vi "Test Multiplexing.vi"() -> ()   [LabVIEW 2015]
uses:
  Typedefs/HRTF-Hardware Config (TDT).ctl
  PXI DAQ VIs/TDT VIs/Typedefs/TDT-Output source.ctl
  PXI DAQ VIs/TDT VIs/Typedefs/TDT-Device ID.ctl
  PXI DAQ VIs/TDT VIs/Typedefs/TDT-Device Config.ctl
  PXI DAQ VIs/TDT VIs/Typedefs/TDT-Input source.ctl
panel:
  in  "read":bool
  out "GetTagVal":sgl
  in  "stop":bool
  in  "Value":u8=255 format="%08b"
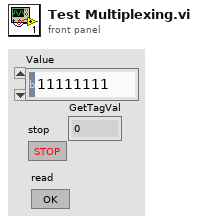
[diagram p1: front panel]
types:
  T1 = typedef "TDT-Device Config.ctl" = cluster{"Output":T2, "Input":T4}
  T2 = typedef "TDT-Output source.ctl" = cluster{"Device":T3, "Num":i32}
  T3 = typedef "TDT-Device ID.ctl" = enum16{"None", "PA5", "RP2", "RL2", "RA16", "RV8", "RX5", "RX6", "RX7", "RX8", "RZ2", "RZ5", "RZ6"}
  T4 = typedef "TDT-Input source.ctl" = enum16{"Front Panel", "RA4LI", "RA16LI"}
  T5 = typedef "HRTF-Hardware Config (TDT).ctl" = cluster{"Output":T2, "Speaker":cluster{"Channel":i32, "Primary mux":i32, "Secondary mux":i32}, "Right mic":i32, "Left mic":i32}
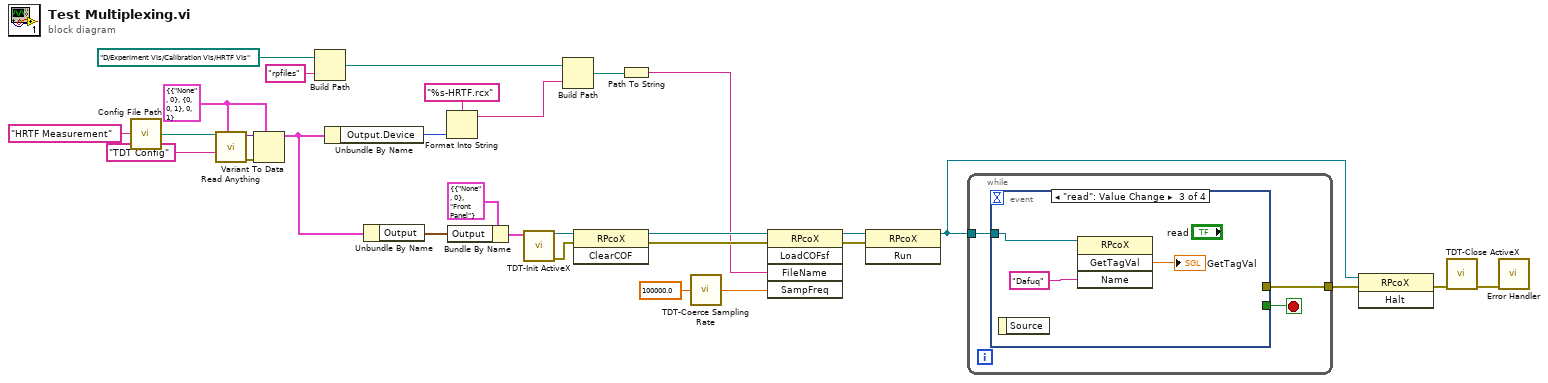
[diagram p0: block diagram]
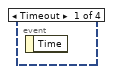
[diagram p2: hidden frame]
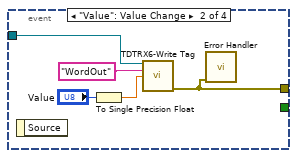
[diagram p3: hidden frame]
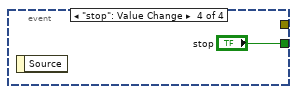
[diagram p4: hidden frame]
diagram:
  w26 = T5 {"Output"={"Device"=enum."None", "Num"=0}, "Speaker"={"Channel"=0, "Primary mux"=0, "Secondary mux"=1}, "Right mic"=0, "Left mic"=1} ("TDT")
  n1 = call "Config File Path.vi"("AppName"="HRTF Measurement") -> ("Default config file name"=w27:path)
  n2 = call "Read Anything.vi"("Type of Anything"=w26, "Section Name (Name of \"Type of Anything\")"="TDT Config" ("Section Name (Name of \"Type of Anything\")"), "Path (dialog)"=w27) -> ("Error Out"=w30:errorcluster, "Anything"=w29:variant)  [unwired: 6 in, 1 out]
  n3 = Variant To Data(error in=w30, type=w26, Variant=w29) -> (data=w21:T5)  [unwired: 1 out]
  n4 = Build Path(base path=path "D:/Experiment VIs/Calibration VIs/HRTF VIs", name or relative path="rpfiles") -> (appended path=w14:path)
  n5 = Unbundle By Name(w21) -> ("Output.Device"=w24:T3)
  n6 = Unbundle By Name(w21) -> ("Output"=w20:T2)
  n7 = Format Into String(format string="%s-HRTF.rcx", w24) -> (resulting string=w12:string)  [unwired: 2 in, 1 out]
  n8 = Bundle By Name(cluster=T1 {"Output"={"Device"=enum."None", "Num"=0}, "Input"=enum."Front Panel"} ("TDT-Device Config"), "Output"=w20) -> (w22:T1)
  n9 = call "TDT-Init ActiveX.vi"("TDT-Device Config"=w22) -> ("RPcox"=w16:refnum<k7>, "error out"=w17:errorcluster)  [unwired: 11 in, 2 out]
  n10 = Build Path(base path=w14, name or relative path=w12) -> (appended path=w13:path)
  n11 = invoke class="RPcoX" method="ClearCOF"(reference=w16, error in=w17) -> (reference out=w19:refnum<k7>, error out=w18:errorcluster)  [unwired: 1 in, 1 out]
  n12 = Path To String(path=w13) -> (string=w11:string)
  n13 = call "TDT-Coerce Sampling Rate.vi"("Fs (Hz)"=100000.0) -> ("Coerced"=w9:dbl)
  n14 = invoke class="RPcoX" method="LoadCOFsf"(reference=w19, error in=w18, "FileName"=w11, "SampFreq"=w9) -> (reference out=w6:refnum<k7>, error out=w5:errorcluster)  [unwired: 1 in, 3 out]
  n15 = invoke class="RPcoX" method="Run"(reference=w6, error in=w5) -> (reference out=w1:refnum<k7>)  [unwired: 1 in, 2 out]
  n16 = while {
    tunnel: [w33] -> w4
    tunnel: w1 -> [w31]
    stop <- w32 stop-if-true
    n17 = event shown="[2] \"read\": Value Change" {
      selector: _ -> [_ _ _ _]
      dyn-events: _ -> [_ _ _ _]
      timeout: _ -> [_ _ _ _]
      tunnel: w31 -> [_ w34 w40 _]
      tunnel: [_ w37 _ _] -> w33
      tunnel: [_ _ _ "stop"] -> w32
      event Timeout {
        n18 = event-data() -> ()  [unwired: 1 in, 1 out]
      }
      event "Value": Value Change {
        n19 = event-data() -> ()  [unwired: 1 in, 1 out]
        n20 = To Single Precision Float(number="Value") -> (single precision float=w35:sgl)
        n21 = call "TDTRX6-Write Tag.vi"("RPcox"=w34, "Name"="WordOut", "Value"=w35) -> ("error out"=w37:errorcluster)  [unwired: 11 in, 1 out]
        n22 = call "Error Handler.vi"("error in (no error)"=w37) -> ()  [unwired: 13 in, 2 out]
      }
      event "read": Value Change {
        n23 = event-data() -> ()  [unwired: 1 in, 1 out]
        n24 = invoke class="RPcoX" method="GetTagVal"(reference=w40, "Name"="Dafuq") -> ("GetTagVal"=→"GetTagVal":sgl)  [unwired: 2 in, 3 out]
      }
      event "stop": Value Change {
        n25 = event-data() -> ()  [unwired: 1 in, 1 out]
      }
    }
  }
  n26 = invoke class="RPcoX" method="Halt"(reference=w1, error in=w4) -> (error out=w3:errorcluster)  [unwired: 1 in, 2 out]
  n27 = call "TDT-Close ActiveX.vi"("error in (no error)"=w3) -> ("error out"=w7:errorcluster)  [unwired: 14 in]
  n28 = call "Error Handler.vi"("error in (no error)"=w7) -> ()  [unwired: 13 in, 2 out]
